vi "Query Voltage Range.vi"() -> ()   [LabVIEW 2015]
panel:
  out "Maximum value":u16
  out "Minimum value":u16
  in  "error in (no error)":errorcluster
  out "VISA resource name out":refnum<visa-resource-name>
  out "error out":errorcluster
  in  "VISA resource name":refnum<visa-resource-name>
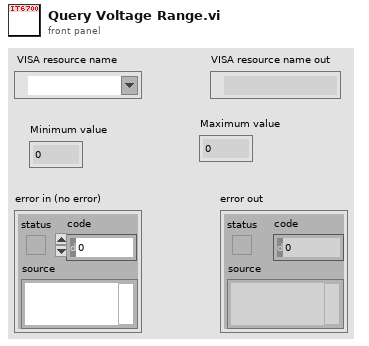
[diagram p1: front panel]
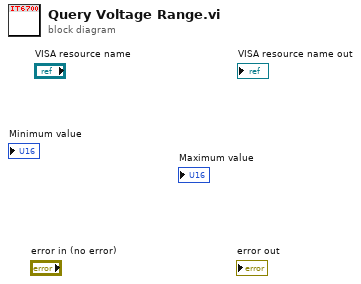
[diagram p0: block diagram]
diagram:
